vi "SR430_transaction.vi"(0 "SR430 VISA Cluster":T1, 2 "SR430 Command String":string, 3 "Bytes to read (1024)":u32=1024, 4 "Read (FALSE)":bool, 5 "error in (no error)":errorcluster, 9 "ignoreInterfaceReady (FALSE)":bool) -> (14 "dup SR430 VISA Cluster":T1, 16 "SR430 Response":string, 17 "bytes read":u32=48, 19 "error out":errorcluster)   [LabVIEW 2015, in "SR430Driver.lvlib"]
doc: "Makes the transaction with the instrument, formating command or query strings.\n\nPlease note, that this transaction-VI is NOT reeentrant, since it is not foreseen to operate more than one device of this type at the same time!\n\n\nCopyright (C) \nGesellschaft f. Schwerionenforschung, GSI\nPlanckstr. 1\n64291 Darmstadt\nGermany\n\nContact: http://www-wnt.gsi.de/labview, d.beck@gsi.de\n\nThis program is free software; you can redistribute it and/or\nmodify it under the terms of the GNU General Public License\nas published by the Free Software Foundation; either version 2\nof the License, or (at your option) any later version.\n\nThis program is distributed in the hope that it will be useful,\nbut WITHOUT ANY WARRANTY; without even the implied warranty of\nMERCHANTABILITY or FITNESS FOR A PARTICULAR PURPOSE. See the\nGNU General Public License for more details (http://www.gnu.org)."
uses:
  SR430Driver.lvlib
  SR430_VISA Control.ctl
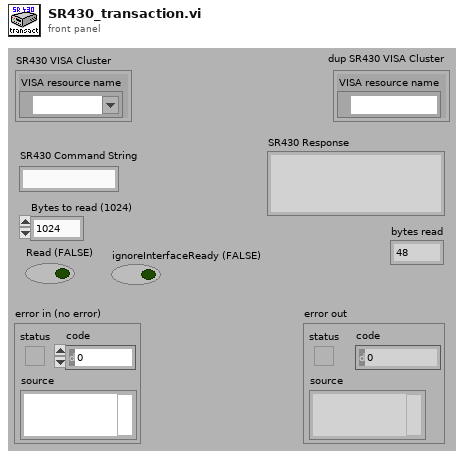
[diagram p1: front panel]
types:
  T1 = typedef "SR430Driver.lvlib/SR430_VISA Control.ctl" = cluster{"VISA resource name":refnum<visa-resource-name>}
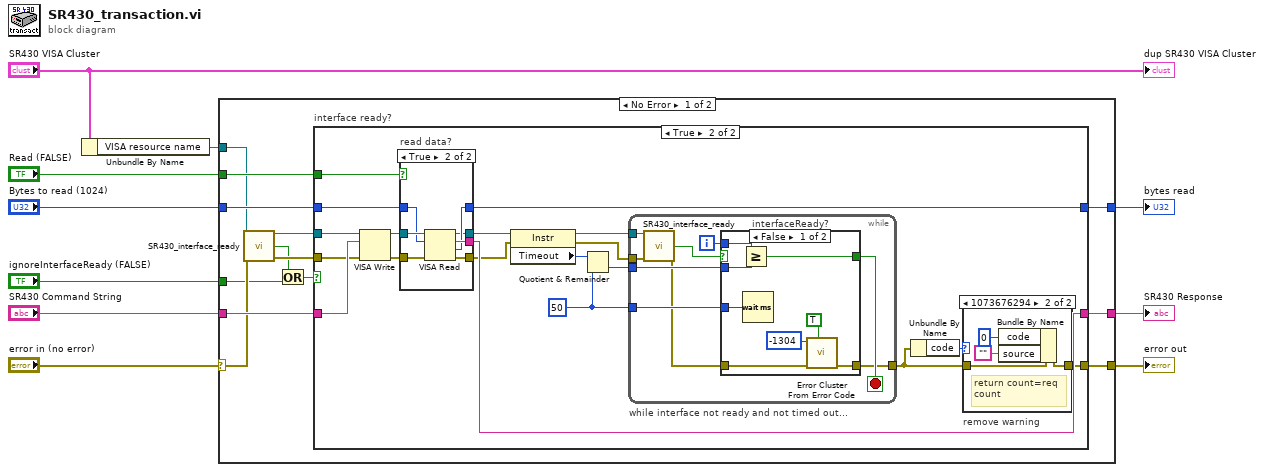
[diagram p0: block diagram]
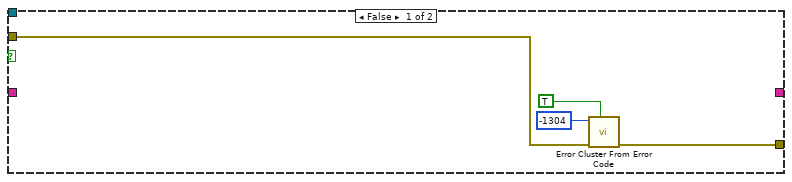
[diagram p2: hidden frame]
diagram:
  n1 = Unbundle By Name("SR430 VISA Cluster") -> ("VISA resource name"=w7:refnum<visa-resource-name>)
  n2 = case shown="No Error" "error in (no error)" {
    selector: "error in (no error)" -> [w14 w80]
    tunnel: w7 -> [w17 _]
    tunnel: [w20 _] -> w6
    tunnel: [w18 w80] -> w9
    tunnel: [w19 _] -> w5
    tunnel: "SR430 Command String" -> [w23 _]
    tunnel: "Read (FALSE)" -> [w22 _]
    tunnel: "Bytes to read (1024)" -> [w21 _]
    tunnel: "ignoreInterfaceReady (FALSE)" -> [w11 _]
    frame No Error {
      n3 = call "SR430_interface_ready.vi"("VISA resource name"=w17, "error in (no error)"=w14) -> ("VISA resource name out"=w16:refnum<visa-resource-name>, "interfaceReady?"=w12:bool, "error out"=w15:errorcluster)  [unwired: 11 in]
      n4 = Or(x=w12, y=w11) -> (x .or. y?=w13:bool)
      n5 = case "interface ready?" shown="True" w13 {
        tunnel: w23 -> [_ w44]
        tunnel: w22 -> [_ w43]
        tunnel: w21 -> [_ w42]
        tunnel: [_ w41] -> w20
        tunnel: [_ w40] -> w19
        tunnel: [w27 w38] -> w18
        tunnel: w16 -> [_ w29]
        tunnel: w15 -> [w24 w28]
        frame False {
          n6 = call <vilib>:"Error Cluster From Error Code.vi"("show call chain? (False)"=TRUE, "error in (no error)"=w24, "error code (0)"=-1304 ("code")) -> ("error out"=w27:errorcluster)  [unwired: 6 in]
        }
        frame True {
          w30 = u32 50 ("y")
          n7 = VISA Write(VISA resource name=w29, write buffer=w44, error in (no error)=w28) -> (VISA resource name out=w45:refnum<visa-resource-name>, error out=w46:errorcluster)  [unwired: 1 out]
          n8 = case "read data?" shown="True" w43 {
            tunnel: w46 -> [w72 w79]
            tunnel: w45 -> [w71 w78]
            tunnel: w42 -> [_ w77]
            tunnel: [_ w76] -> w41
            tunnel: [w72 w75] -> w36
            tunnel: [_ w74] -> w40
            tunnel: [w71 w73] -> w37
            frame False {
            }
            frame True {
              n9 = VISA Read(VISA resource name=w78, byte count=w77, error in (no error)=w79) -> (VISA resource name out=w73:refnum<visa-resource-name>, read buffer=w76:string, return count=w74:u32, error out=w75:errorcluster)
            }
          }
          n10 = property on="Property Node" class="Instr"(reference=w37, error in=w36) -> (reference out=w34:refnum<visa-resource-name>, error out=w35:errorcluster, "Timeout"=w32:u32)
          n11 = Quotient & Remainder(x=w32, y=w30) -> (floor(x/y)=w31:u32)  [unwired: 1 out]
          n12 = while "while interface not ready and not timed out..." {
            tunnel: [w47] -> w33
            tunnel: w35 -> [w55]
            tunnel: w34 -> [w54]
            tunnel: w31 -> [w51]
            tunnel: w30 -> [w49]
            i -> [w50]
            stop <- w52 stop-if-true
            n13 = call "SR430_interface_ready.vi"("VISA resource name"=w54, "error in (no error)"=w55) -> ("interfaceReady?"=w53:bool, "error out"=w48:errorcluster)  [unwired: 11 in, 1 out]
            n14 = case "interfaceReady?" shown="False" w53 {
              selector: w53 -> [_ w65]
              tunnel: [w61 w65] -> w52
              tunnel: w51 -> [w63 _]
              tunnel: w50 -> [w62 _]
              tunnel: w49 -> [w60 _]
              tunnel: [w57 w64] -> w47
              tunnel: w48 -> [w58 w64]
              frame False {
                n15 = Greater Or Equal?(x=w62, y=w63) -> (x >= y?=w61:bool)
                n16 = Wait (ms)(milliseconds to wait=w60) -> ()  [unwired: 1 out]
                n17 = call <vilib>:"Error Cluster From Error Code.vi"("show call chain? (False)"=TRUE, "error in (no error)"=w58, "error code (0)"=-1304 ("code")) -> ("error out"=w57:errorcluster)  [unwired: 6 in]
              }
              frame True {
              }
            }
          }
          n18 = Unbundle By Name(w33) -> ("code"=w39:i32)
          n19 = case "remove warning" shown="1073676294" w39 {
            tunnel: w33 -> [w66 w70]
            tunnel: [w66 w69] -> w38
            frame 0, Default {
            }
            frame 1073676294 {
              # "return count=req\ncount"
              n20 = Bundle By Name(cluster=w70, "code"=0, "source"="") -> (w69:errorcluster)
            }
          }
        }
      }
    }
    frame Error {
    }
  }
  "SR430 Response" <- w6
  "error out" <- w9
  "bytes read" <- w5
  "dup SR430 VISA Cluster" <- "SR430 VISA Cluster"
